vi "Demo - Initialise Setting for Hardware in the Loop.vi"(9 "Analog In Data Size":T1, 10 "Samples to Read":i32, 11 "Address":string) -> (0 "error out":errorcluster, 2 "Ready":bool)   [LabVIEW 2017]
uses:
  Communications/Typedefs/Data Size--Enum.ctl
  Communications/Communications Library.lvlib
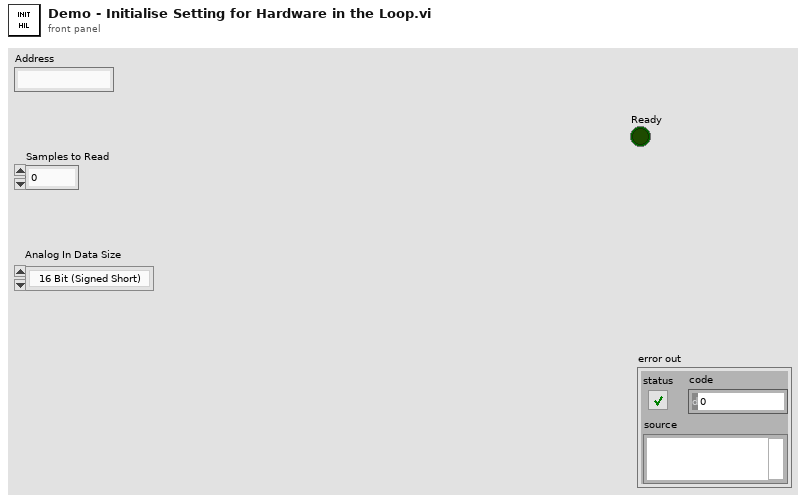
[diagram p1: front panel]
types:
  T1 = typedef "Communications Library.lvlib/Data Size--Enum.ctl" = enum16{"16 Bit (Signed Short)", "32 Bit (Signed Long)"}
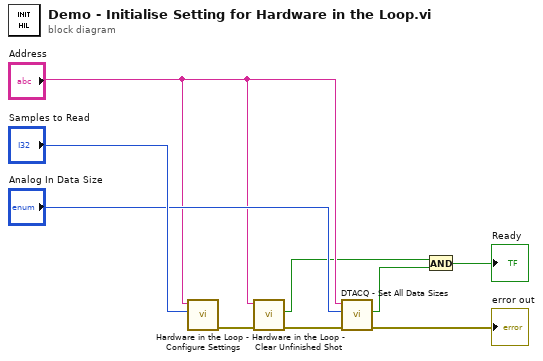
[diagram p0: block diagram]
diagram:
  n1 = call "Hardware in the Loop - Configure Settings.vi"("Samples to Read"="Samples to Read", "Address"="Address") -> ("error out"=w7:errorcluster)  [unwired: 9 in]
  n2 = call "Hardware in the Loop - Clear Unfinished Shot.vi"("error in"=w7, "Address"="Address") -> ("error out"=w8:errorcluster, "Ready"=w2:bool)  [unwired: 8 in]
  n3 = call "DTACQ - Set All Data Sizes.vi"("error in"=w8, "Analog In Data Size"="Analog In Data Size", "Address"="Address") -> ("error out"=→"error out":errorcluster, "Acknowledged"=w3:bool)  [unwired: 7 in]
  n4 = And(x=w2, y=w3) -> (x .and. y?=→"Ready":bool)
